vi "Create Test Channels.vi"(8 "error in":errorcluster) -> (0 "error out":errorcluster, 3 "CIFCorePlugin out":refnum<class "CIFCorePlugin.lvclass">)   [LabVIEW 2021, in "Template Test Helpers.lvlib"]
uses:
  Template Test Helpers.lvlib
  Common/Template_Common.lvlib
  <vilib>/CIF Foundation/CIF Core/CIFCore/Class/CIFCorePlugin.lvclass
  <vilib>/CIF Foundation/CIF Channels Core/CIFChannels/CIFChannels.lvclass
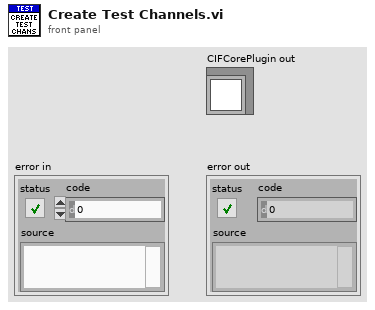
[diagram p1: front panel]
types:
  T1 = typedef "ChannelRegistrar.lvlib/Channel Definition.ctl" = cluster{"Name":string, "Direction":T2, "Type":T3, "Custom Config Data":u8[]}
  T2 = typedef "CIFChannels.lvclass/Direction.ctl" = enum16{"Publisher", "Subscriber"}
  T3 = typedef "ChannelRegistrar.lvlib/Registered Channel Types.ctl" = enum16{"Custom", "Double_Tag", "I64_Tag", "U64_Tag", "U8_FIFO", "CAN_FIFO", "L2Enet_FIFO", "DAQ_FIFO", "Universal_FIFO", "String_Tag"}
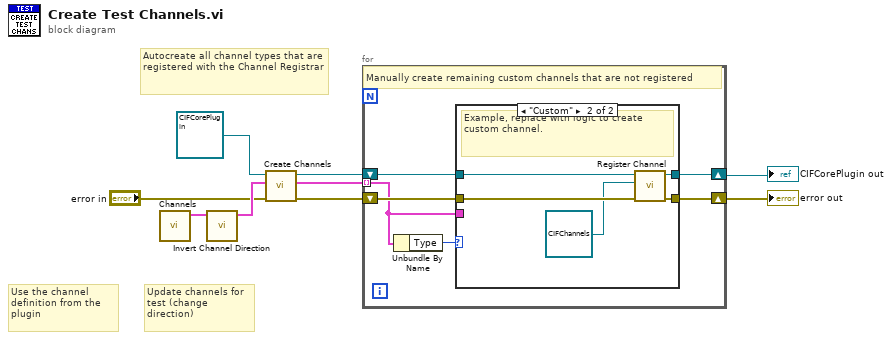
[diagram p0: block diagram]
diagram:
  # "Update channels for test (change direction)"
  # "Use the channel definition from the plugin"
  # "Autocreate all channel types that are registered with the Channel Registrar"
  n1 = call "Channels.vi"() -> ("Channels to Create"=w8:T1[])  [unwired: 10 in, 1 out]
  n2 = call "Invert Channel Direction.vi"("Channels to Create"=w8) -> ("Inverted Channels to Create"=w9:T1[])  [unwired: 10 in]
  n3 = call <vilib>:"Create Channels.vi"("error in (no error)"="error in", "Channels to Create in"=w9, "CIFCorePlugin in"=refnum<class "CIFCorePlugin.lvclass"> refnum) -> ("error out"=w4:errorcluster, "Channels to Create out"=w2:T1[], "CIFCorePlugin out"=w3:refnum<class "CIFCorePlugin.lvclass">)  [unwired: 6 in]
  n4 = for {
    tunnel: w2 -> [w10] mode=indexing
    shift-right: [w13] -> w7
    shift-left: w3 -> [w15]
    shift-right: [w12] -> w5
    shift-left: w4 -> [w14]
    # "Manually create remaining custom channels that are not registered"
    n5 = Unbundle By Name(w10) -> ("Type"=w11:T3)
    n6 = case shown="\"Custom\"" w11 {
      tunnel: w15 -> [w17 w22]
      tunnel: w14 -> [w16 w21]
      tunnel: [w17 w20] -> w13
      tunnel: [w16 w19] -> w12
      tunnel: w10 -> [_ _]
      frame Default {
      }
      frame "Custom" {
        # "Example, replace with logic to create custom channel."
        n7 = call <vilib>:"Register Channel.vi"("error in (no error)"=w21, "Channel"=refnum<class "CIFChannels.lvclass"> refnum, "CIFCorePlugin in"=w22) -> ("error out"=w19:errorcluster, "CIFCorePlugin out"=w20:refnum<class "CIFCorePlugin.lvclass">)  [unwired: 7 in]
      }
    }
  }
  "CIFCorePlugin out" <- w7
  "error out" <- w5
